vi "Supervisor Read Client.vi"() -> ()   [LabVIEW 2017]
uses:
  <vilib>/OPCUA/controls/NodeIds.ctl
  <vilib>/OPCUA/controls/NodeId.ctl
  <vilib>/OPCUA/NI OPC UA Client.lvlib
panel:
  in  "stop":bool
  out "error out":errorcluster
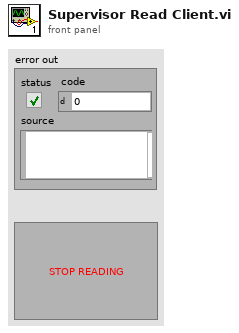
[diagram p1: front panel]
types:
  T1 = cluster{"message mode":enum16{"None", "Sign", "Sign and Encrypt"}, "security":enum16{"Basic256", "Basic128Rsa15"}}
  T2 = typedef "NodeIds.ctl" = T3[]
  T3 = typedef "NodeId.ctl" = string
  T4 = typedef "OPC UA Client Refnum.ctl" = refnum<k21>
  T5 = typedef "Subscription ID.ctl" = u32
  T6 = typedef "Subscription Data Change.ctl" = cluster{"node ID":T3, " value":variant, "timestamp":timestamp, "data type":T7, "status code":T8}
  T7 = typedef "Data Type.ctl" = u16
  T8 = typedef "OPC UA StatusCode.ctl" = u32
  T9 = cluster{"[0]":sgl, "[1]":sgl, "[2]":sgl, "[3]":sgl, "[4]":sgl, "[5]":sgl, "[6]":sgl, "[7]":sgl, "[8]":sgl, "[9]":sgl, "[10]":sgl, "[11]":sgl, "[12]":sgl, "[13]":sgl, "[14]":sgl, "[15]":sgl, "[16]":sgl, "[17]":sgl, "[18]":sgl, "[19]":sgl, "[20]":sgl, "[21]":sgl, "[22]":sgl, "[23]":sgl, "[24]":sgl, "[25]":sgl, "[26]":sgl, "[27]":sgl, "[28]":sgl, "[29]":sgl, "[30]":sgl, "[31]":sgl, "[32]":sgl, "[33]":sgl, "[34]":sgl, "[35]":sgl, "[36]":sgl, "[37]":sgl, "[38]":sgl, "[39]":sgl, "[40]":sgl, "[41]":sgl, "[42]":sgl, "[43]":sgl, "[44]":sgl, "[45]":sgl, "[46]":sgl, "[47]":sgl, "[48]":sgl, "[49]":sgl, "[50]":sgl, "[51]":sgl, "[52]":sgl, "[53]":sgl, "[54]":sgl, "[55]":sgl, "[56]":sgl, "[57]":sgl, "[58]":sgl, "[59]":sgl, "[60]":sgl, "[61]":sgl, "[62]":sgl}
  T10 = cluster{"[0]":sgl, "[1]":sgl, "[2]":sgl, "[3]":sgl, "[4]":sgl, "[5]":sgl, "[6]":sgl, "[7]":sgl, "[8]":sgl, "[9]":sgl}
  T11 = cluster{"[0]":bool, "[1]":bool, "[2]":bool, "[3]":bool, "[4]":bool, "[5]":bool, "[6]":bool, "[7]":bool, "[8]":bool, "[9]":bool, "[10]":bool, "[11]":bool, "[12]":bool, "[13]":bool, "[14]":bool, "[15]":bool, "[16]":bool, "[17]":bool, "[18]":bool, "[19]":bool, "[20]":bool, "[21]":bool, "[22]":bool, "[23]":bool, "[24]":bool, "[25]":bool, "[26]":bool, "[27]":bool, "[28]":bool, "[29]":bool, "[30]":bool, "[31]":bool, "[32]":bool, "[33]":bool, "[34]":bool, "[35]":bool, "[36]":bool, "[37]":bool, "[38]":bool, "[39]":bool, "[40]":bool, "[41]":bool, "[42]":bool, "[43]":bool, "[44]":bool, "[45]":bool, "[46]":bool, "[47]":bool, "[48]":bool, "[49]":bool, "[50]":bool, "[51]":bool, "[52]":bool, "[53]":bool, "[54]":bool, "[55]":bool, "[56]":bool, "[57]":bool, "[58]":bool, "[59]":bool, "[60]":bool, "[61]":bool, "[62]":bool}
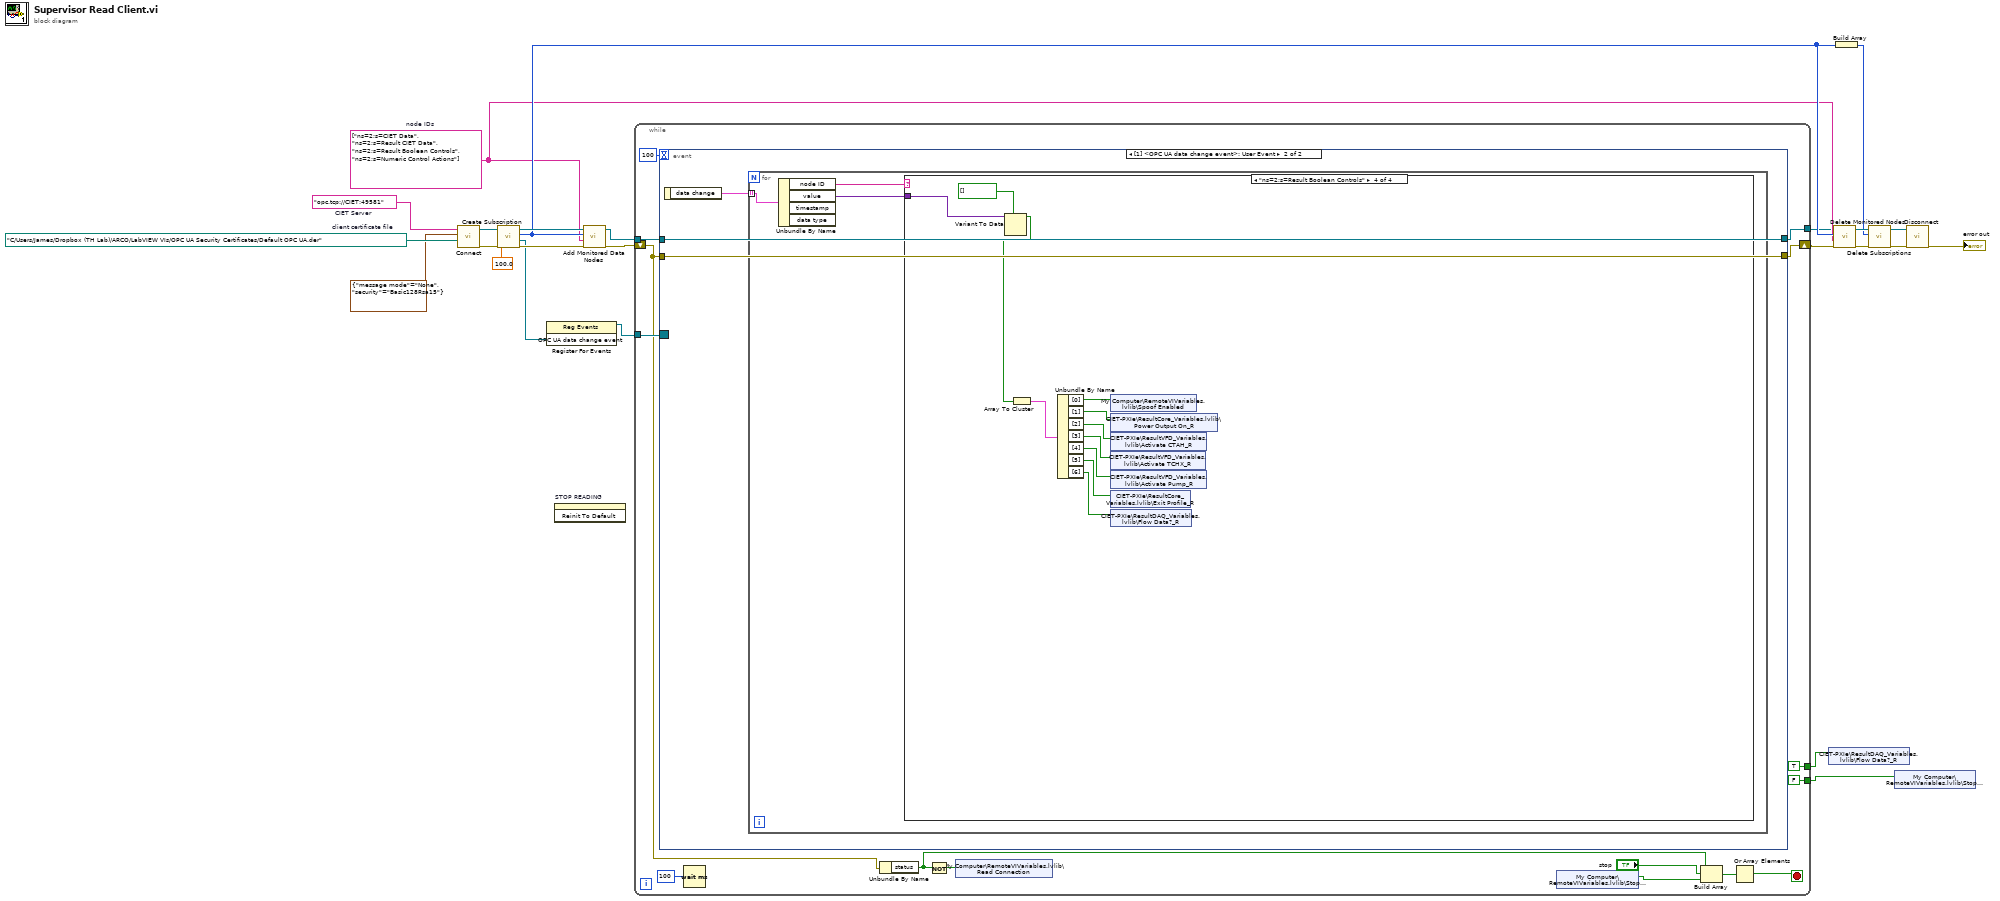
[diagram p0: block diagram]
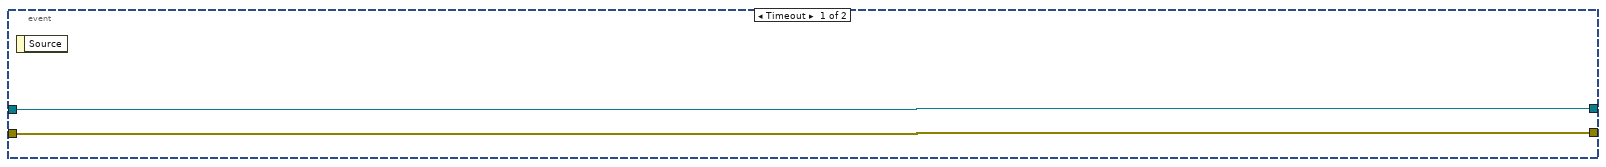
[diagram p2: hidden frame]
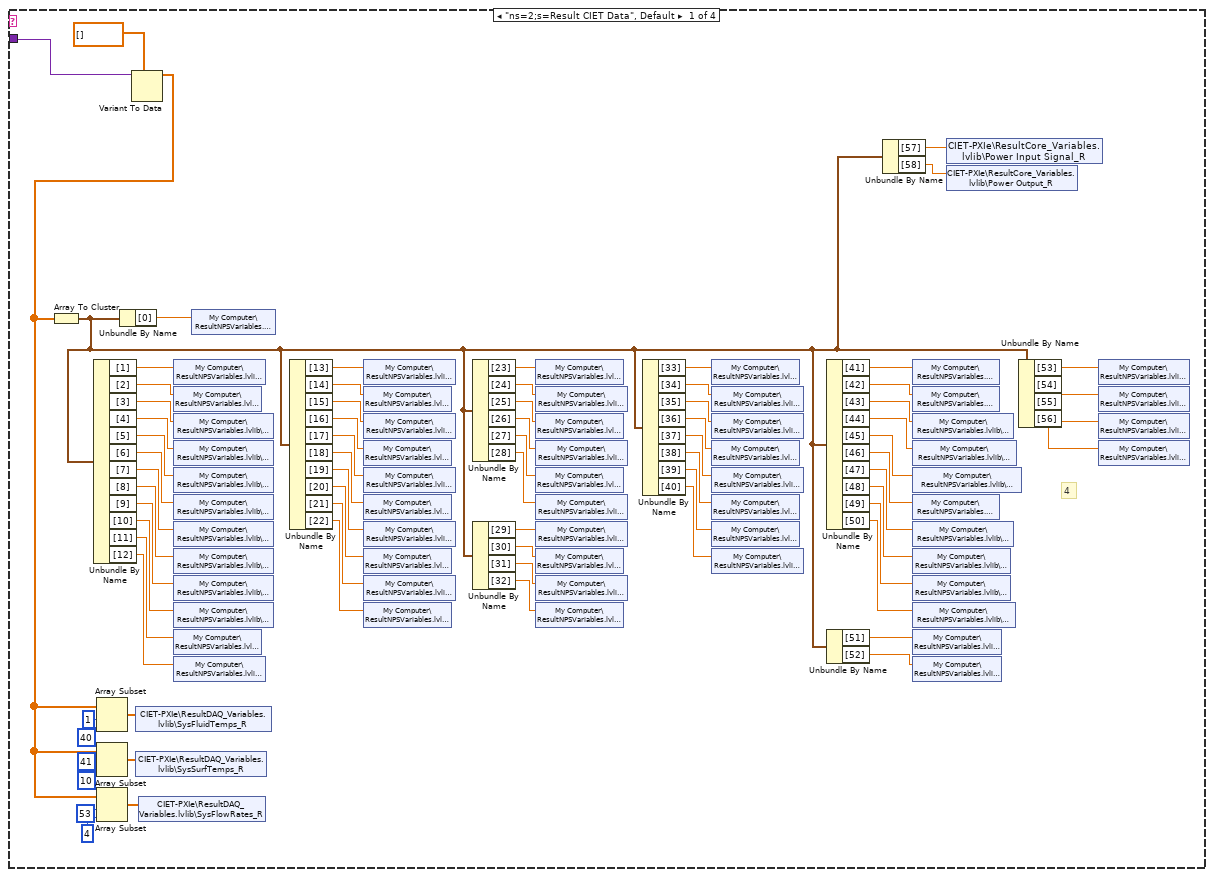
[diagram p3: hidden frame]
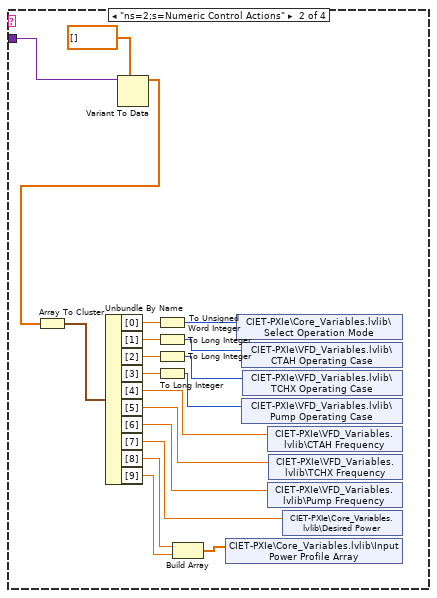
[diagram p4: hidden frame]
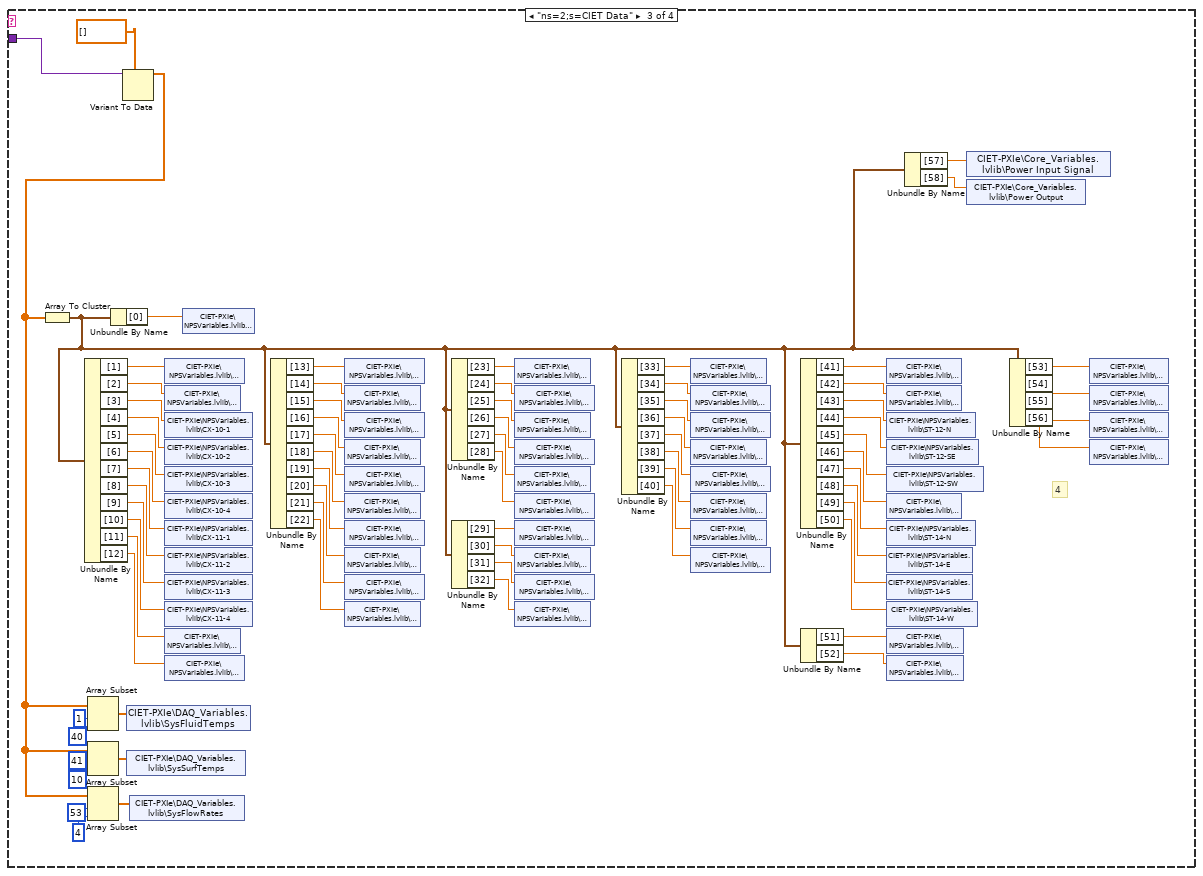
[diagram p5: hidden frame]
diagram:
  w7 = T2 ["ns=2;s=CIET Data", "ns=2;s=Result CIET Data", "ns=2;s=Result Boolean Controls", "ns=2;s=Numeric Control Actions"]  # node IDs
  w22 = path "C:/Users/James/Dropbox (TH Lab)/ARCO/LabVIEW VIs/OPC UA Security Certificates/Default OPC UA.der"  # client certificate file
  w23 = "opc.tcp://CIET:49581"  # CIET Server
  n1 = call <vilib>:"Connect.vi"("client certificate file"=w22, "security policy"=T1 {"message mode"=enum."None", "security"=enum."Basic128Rsa15"}, "server endpoint URL"=w23) -> ("error out"=w3:errorcluster, "OPC UA client refnum out"=w20:T4)  [unwired: 6 in, 1 out]
  n2 = call <vilib>:"Create Subscription.vi"("error in (no error)"=w3, "publishing interval (1000 ms)"=100.0, "OPC UA client refnum in"=w20) -> ("error out"=w18:errorcluster, "OPC UA data change event"=w17:refnum<user-event>, "subscription ID out"=w12:T5, "OPC UA client refnum out"=w19:T4)  [unwired: 4 in, 1 out]
  n3 = register-events(w17) -> (reference out=w10:refnum<event-registration>)  [unwired: 2 in, 1 out]
  n4 = invoke on="STOP READING" class="Bool" method="Reinit To Default"() -> ()  [unwired: 3 in, 3 out]
  n5 = call <vilib>:"Add Monitored Data Nodes.vi"("error in (no error)"=w18, "node IDs"=w7, "subscription ID in"=w12, "OPC UA client refnum in"=w19) -> ("error out"=w8:errorcluster, "OPC UA client refnum out"=w9:T4)  [unwired: 4 in, 2 out]
  n6 = while {
    tunnel: w10 -> [w39]
    tunnel: w9 -> [w38]
    tunnel: [w37] -> w6
    tunnel: [FALSE] -> w4
    shift-right: [w33] -> w2
    shift-left: w8 -> [w32]
    tunnel: [TRUE ("Flow Data?_R")] -> w1
    stop <- w31 stop-if-true
    n7 = event shown="[1] <OPC UA data change event>: User Event" {
      selector: w39 -> [_ _]
      dyn-events: _ -> [_ _]
      timeout: 100 -> [_ _]
      tunnel: w38 -> [w41 w44]
      tunnel: [w41 w44] -> w37
      tunnel: w32 -> [w40 w43]
      tunnel: [w40 w43] -> w33
      event Timeout {
        n8 = event-data() -> ()  [unwired: 1 in, 1 out]
      }
      event User Event {
        n9 = event-data() -> ("data change"=w42:T6[])  [unwired: 1 in]
        n10 = for {
          tunnel: w42 -> [w47] mode=indexing
          n11 = Unbundle By Name(w47) -> ("node ID"=w46:T3, "value"=w45:variant)  [unwired: 2 out]
          n12 = case shown="\"ns=2;s=Result Boolean Controls\"" w46 {
            tunnel: w45 -> [w53 w136 w151 w221]
            frame "ns=2;s=Result CIET Data", Default {
              # "4"
              n13 = Variant To Data(type=sgl[] [], Variant=w53) -> (data=w52:sgl[])  [unwired: 1 in, 1 out]
              n14 = Array To Cluster(array=w52) -> (cluster=w50:T9)
              n15 = Unbundle By Name(w50) -> ("[1]"=w60:sgl, "[2]"=w62:sgl, "[3]"=w63:sgl, "[4]"=w64:sgl, "[5]"=w65:sgl, "[6]"=w66:sgl, "[7]"=w67:sgl, "[8]"=w68:sgl, "[9]"=w69:sgl, "[10]"=w70:sgl, "[11]"=w71:sgl, "[12]"=w72:sgl)
              n16 = Array Subset(array=w52, index=1, length=40) -> (w117:sgl[])
              n17 = Array Subset(array=w52, index=41, length=10) -> (w118:sgl[])
              n18 = Array Subset(array=w52, index=53, length=4) -> (w119:sgl[])
              n19 = Unbundle By Name(w50) -> ("[0]"=w61:sgl)
              n20 = shared-variable "CIET-PXIe\\ResultDAQ_Variables.lvlib\\SysFluidTemps_R"(w117) -> ()  [unwired: 1 in, 1 out]
              n21 = shared-variable "CIET-PXIe\\ResultDAQ_Variables.lvlib\\SysSurfTemps_R"(w118) -> ()  [unwired: 1 in, 1 out]
              n22 = shared-variable "CIET-PXIe\\ResultDAQ_Variables.lvlib\\SysFlowRates_R"(w119) -> ()  [unwired: 1 in, 1 out]
              n23 = shared-variable "My Computer\\ResultNPSVariables.lvlib\\WT-10_R"(w60) -> ()  [unwired: 1 in, 1 out]
              n24 = shared-variable "My Computer\\ResultNPSVariables.lvlib\\BT-11_R"(w62) -> ()  [unwired: 1 in, 1 out]
              n25 = shared-variable "My Computer\\ResultNPSVariables.lvlib\\CX-10-1_R"(w63) -> ()  [unwired: 1 in, 1 out]
              n26 = shared-variable "My Computer\\ResultNPSVariables.lvlib\\CX-10-2_R"(w64) -> ()  [unwired: 1 in, 1 out]
              n27 = shared-variable "My Computer\\ResultNPSVariables.lvlib\\CX-10-3_R"(w65) -> ()  [unwired: 1 in, 1 out]
              n28 = shared-variable "My Computer\\ResultNPSVariables.lvlib\\CX-10-4_R"(w66) -> ()  [unwired: 1 in, 1 out]
              n29 = shared-variable "My Computer\\ResultNPSVariables.lvlib\\CX-11-1_R"(w67) -> ()  [unwired: 1 in, 1 out]
              n30 = shared-variable "My Computer\\ResultNPSVariables.lvlib\\CX-11-2_R"(w68) -> ()  [unwired: 1 in, 1 out]
              n31 = shared-variable "My Computer\\ResultNPSVariables.lvlib\\CX-11-3_R"(w69) -> ()  [unwired: 1 in, 1 out]
              n32 = shared-variable "My Computer\\ResultNPSVariables.lvlib\\CX-11-4_R"(w70) -> ()  [unwired: 1 in, 1 out]
              n33 = shared-variable "My Computer\\ResultNPSVariables.lvlib\\BT-12_R"(w71) -> ()  [unwired: 1 in, 1 out]
              n34 = shared-variable "My Computer\\ResultNPSVariables.lvlib\\WT-13_R"(w72) -> ()  [unwired: 1 in, 1 out]
              n35 = shared-variable "My Computer\\ResultNPSVariables.lvlib\\Time_R"(w61) -> ()  [unwired: 1 in, 1 out]
              n36 = Unbundle By Name(w50) -> ("[13]"=w73:sgl, "[14]"=w74:sgl, "[15]"=w75:sgl, "[16]"=w76:sgl, "[17]"=w77:sgl, "[18]"=w78:sgl, "[19]"=w79:sgl, "[20]"=w80:sgl, "[21]"=w81:sgl, "[22]"=w82:sgl)
              n37 = shared-variable "My Computer\\ResultNPSVariables.lvlib\\WT-20_R"(w73) -> ()  [unwired: 1 in, 1 out]
              n38 = shared-variable "My Computer\\ResultNPSVariables.lvlib\\BT-21_R"(w74) -> ()  [unwired: 1 in, 1 out]
              n39 = shared-variable "My Computer\\ResultNPSVariables.lvlib\\WT-22_R"(w75) -> ()  [unwired: 1 in, 1 out]
              n40 = shared-variable "My Computer\\ResultNPSVariables.lvlib\\BT-23_R"(w76) -> ()  [unwired: 1 in, 1 out]
              n41 = shared-variable "My Computer\\ResultNPSVariables.lvlib\\WT-24_R"(w77) -> ()  [unwired: 1 in, 1 out]
              n42 = shared-variable "My Computer\\ResultNPSVariables.lvlib\\BT-25_R"(w78) -> ()  [unwired: 1 in, 1 out]
              n43 = shared-variable "My Computer\\ResultNPSVariables.lvlib\\WT-26_R"(w79) -> ()  [unwired: 1 in, 1 out]
              n44 = shared-variable "My Computer\\ResultNPSVariables.lvlib\\BT-27_R"(w80) -> ()  [unwired: 1 in, 1 out]
              n45 = shared-variable "My Computer\\ResultNPSVariables.lvlib\\WT-28_R"(w81) -> ()  [unwired: 1 in, 1 out]
              n46 = shared-variable "My Computer\\ResultNPSVariables.lvlib\\BT-29_R"(w82) -> ()  [unwired: 1 in, 1 out]
              n47 = Unbundle By Name(w50) -> ("[23]"=w83:sgl, "[24]"=w84:sgl, "[25]"=w85:sgl, "[26]"=w86:sgl, "[27]"=w87:sgl, "[28]"=w88:sgl)
              n48 = Unbundle By Name(w50) -> ("[29]"=w89:sgl, "[30]"=w90:sgl, "[31]"=w91:sgl, "[32]"=w92:sgl)
              n49 = shared-variable "My Computer\\ResultNPSVariables.lvlib\\BT-30_R"(w83) -> ()  [unwired: 1 in, 1 out]
              n50 = shared-variable "My Computer\\ResultNPSVariables.lvlib\\WT-31_R"(w84) -> ()  [unwired: 1 in, 1 out]
              n51 = shared-variable "My Computer\\ResultNPSVariables.lvlib\\BT-32_R"(w85) -> ()  [unwired: 1 in, 1 out]
              n52 = shared-variable "My Computer\\ResultNPSVariables.lvlib\\WT-33_R"(w86) -> ()  [unwired: 1 in, 1 out]
              n53 = shared-variable "My Computer\\ResultNPSVariables.lvlib\\BT-34_R"(w87) -> ()  [unwired: 1 in, 1 out]
              n54 = shared-variable "My Computer\\ResultNPSVariables.lvlib\\WT-35_R"(w88) -> ()  [unwired: 1 in, 1 out]
              n55 = shared-variable "My Computer\\ResultNPSVariables.lvlib\\WT-40_R"(w89) -> ()  [unwired: 1 in, 1 out]
              n56 = shared-variable "My Computer\\ResultNPSVariables.lvlib\\BT-41_R"(w90) -> ()  [unwired: 1 in, 1 out]
              n57 = shared-variable "My Computer\\ResultNPSVariables.lvlib\\WT-42_R"(w91) -> ()  [unwired: 1 in, 1 out]
              n58 = shared-variable "My Computer\\ResultNPSVariables.lvlib\\BT-43_R"(w92) -> ()  [unwired: 1 in, 1 out]
              n59 = Unbundle By Name(w50) -> ("[33]"=w93:sgl, "[34]"=w94:sgl, "[35]"=w95:sgl, "[36]"=w96:sgl, "[37]"=w97:sgl, "[38]"=w98:sgl, "[39]"=w99:sgl, "[40]"=w100:sgl)
              n60 = shared-variable "My Computer\\ResultNPSVariables.lvlib\\BT-60_R"(w93) -> ()  [unwired: 1 in, 1 out]
              n61 = shared-variable "My Computer\\ResultNPSVariables.lvlib\\WT-61_R"(w94) -> ()  [unwired: 1 in, 1 out]
              n62 = shared-variable "My Computer\\ResultNPSVariables.lvlib\\WT-62_R"(w95) -> ()  [unwired: 1 in, 1 out]
              n63 = shared-variable "My Computer\\ResultNPSVariables.lvlib\\BT-63_R"(w96) -> ()  [unwired: 1 in, 1 out]
              n64 = shared-variable "My Computer\\ResultNPSVariables.lvlib\\WT-64_R"(w97) -> ()  [unwired: 1 in, 1 out]
              n65 = shared-variable "My Computer\\ResultNPSVariables.lvlib\\BT-65_R"(w98) -> ()  [unwired: 1 in, 1 out]
              n66 = shared-variable "My Computer\\ResultNPSVariables.lvlib\\BT-66_R"(w99) -> ()  [unwired: 1 in, 1 out]
              n67 = shared-variable "My Computer\\ResultNPSVariables.lvlib\\WT-67_R"(w100) -> ()  [unwired: 1 in, 1 out]
              n68 = Unbundle By Name(w50) -> ("[41]"=w101:sgl, "[42]"=w102:sgl, "[43]"=w103:sgl, "[44]"=w104:sgl, "[45]"=w105:sgl, "[46]"=w106:sgl, "[47]"=w107:sgl, "[48]"=w108:sgl, "[49]"=w109:sgl, "[50]"=w110:sgl)
              n69 = Unbundle By Name(w50) -> ("[51]"=w111:sgl, "[52]"=w112:sgl)
              n70 = Unbundle By Name(w50) -> ("[57]"=w49:sgl, "[58]"=w48:sgl)
              n71 = shared-variable "My Computer\\ResultNPSVariables.lvlib\\ST-10_R"(w101) -> ()  [unwired: 1 in, 1 out]
              n72 = shared-variable "My Computer\\ResultNPSVariables.lvlib\\ST-11_R"(w102) -> ()  [unwired: 1 in, 1 out]
              n73 = shared-variable "My Computer\\ResultNPSVariables.lvlib\\ST-12-N_R"(w103) -> ()  [unwired: 1 in, 1 out]
              n74 = shared-variable "My Computer\\ResultNPSVariables.lvlib\\ST-12-SE_R"(w104) -> ()  [unwired: 1 in, 1 out]
              n75 = shared-variable "My Computer\\ResultNPSVariables.lvlib\\ST-12-SW_R"(w105) -> ()  [unwired: 1 in, 1 out]
              n76 = shared-variable "My Computer\\ResultNPSVariables.lvlib\\ST-13_R"(w106) -> ()  [unwired: 1 in, 1 out]
              n77 = shared-variable "My Computer\\ResultNPSVariables.lvlib\\ST-14-N_R"(w107) -> ()  [unwired: 1 in, 1 out]
              n78 = shared-variable "My Computer\\ResultNPSVariables.lvlib\\ST-14-E_R"(w108) -> ()  [unwired: 1 in, 1 out]
              n79 = shared-variable "My Computer\\ResultNPSVariables.lvlib\\ST-14-S_R"(w109) -> ()  [unwired: 1 in, 1 out]
              n80 = shared-variable "My Computer\\ResultNPSVariables.lvlib\\ST-14-W_R"(w110) -> ()  [unwired: 1 in, 1 out]
              n81 = shared-variable "My Computer\\ResultNPSVariables.lvlib\\AT-01_R"(w111) -> ()  [unwired: 1 in, 1 out]
              n82 = shared-variable "My Computer\\ResultNPSVariables.lvlib\\AT-02_R"(w112) -> ()  [unwired: 1 in, 1 out]
              n83 = shared-variable "CIET-PXIe\\ResultCore_Variables.lvlib\\Power Input Signal_R"(w49) -> ()  [unwired: 1 in, 1 out]
              n84 = shared-variable "CIET-PXIe\\ResultCore_Variables.lvlib\\Power Output_R"(w48) -> ()  [unwired: 1 in, 1 out]
              n85 = Unbundle By Name(w50) -> ("[53]"=w113:sgl, "[54]"=w114:sgl, "[55]"=w115:sgl, "[56]"=w116:sgl)
              n86 = shared-variable "My Computer\\ResultNPSVariables.lvlib\\FM-20_R"(w113) -> ()  [unwired: 1 in, 1 out]
              n87 = shared-variable "My Computer\\ResultNPSVariables.lvlib\\FM-30_R"(w114) -> ()  [unwired: 1 in, 1 out]
              n88 = shared-variable "My Computer\\ResultNPSVariables.lvlib\\FM-40_R"(w115) -> ()  [unwired: 1 in, 1 out]
              n89 = shared-variable "My Computer\\ResultNPSVariables.lvlib\\FM-60_R"(w116) -> ()  [unwired: 1 in, 1 out]
            }
            frame "ns=2;s=Numeric Control Actions" {
              n90 = Variant To Data(type=sgl[] [], Variant=w136) -> (data=w138:sgl[])  [unwired: 1 in, 1 out]
              n91 = Array To Cluster(array=w138) -> (cluster=w137:T10)
              n92 = Unbundle By Name(w137) -> ("[0]"=w134:sgl, "[1]"=w133:sgl, "[2]"=w132:sgl, "[3]"=w131:sgl, "[4]"=w126:sgl, "[5]"=w125:sgl, "[6]"=w124:sgl, "[7]"=w123:sgl, "[8]"=w121:sgl, "[9]"=w120:sgl)
              n93 = To Unsigned Word Integer(number=w134) -> (unsigned 16bit integer=w130:u16)
              n94 = To Long Integer(number=w133) -> (32bit integer=w129:i32)
              n95 = To Long Integer(number=w132) -> (32bit integer=w128:i32)
              n96 = To Long Integer(number=w131) -> (32bit integer=w127:i32)
              n97 = Build Array(w121, w120) -> (w122:sgl[])
              n98 = shared-variable "CIET-PXIe\\Core_Variables.lvlib\\Input Power Profile Array"(w122) -> ()  [unwired: 1 in, 1 out]
              n99 = shared-variable "CIET-PXIe\\Core_Variables.lvlib\\Select Operation Mode"(w130) -> ()  [unwired: 1 in, 1 out]
              n100 = shared-variable "CIET-PXIe\\VFD_Variables.lvlib\\CTAH Operating Case"(w129) -> ()  [unwired: 1 in, 1 out]
              n101 = shared-variable "CIET-PXIe\\VFD_Variables.lvlib\\Pump Operating Case"(w127) -> ()  [unwired: 1 in, 1 out]
              n102 = shared-variable "CIET-PXIe\\VFD_Variables.lvlib\\TCHX Operating Case"(w128) -> ()  [unwired: 1 in, 1 out]
              n103 = shared-variable "CIET-PXIe\\VFD_Variables.lvlib\\CTAH Frequency"(w126) -> ()  [unwired: 1 in, 1 out]
              n104 = shared-variable "CIET-PXIe\\VFD_Variables.lvlib\\Pump Frequency"(w124) -> ()  [unwired: 1 in, 1 out]
              n105 = shared-variable "CIET-PXIe\\VFD_Variables.lvlib\\TCHX Frequency"(w125) -> ()  [unwired: 1 in, 1 out]
              n106 = shared-variable "CIET-PXIe\\Core_Variables.lvlib\\Desired Power"(w123) -> ()  [unwired: 1 in, 1 out]
            }
            frame "ns=2;s=CIET Data" {
              # "4"
              n107 = Variant To Data(type=sgl[] [], Variant=w151) -> (data=w148:sgl[])  [unwired: 1 in, 1 out]
              n108 = Array To Cluster(array=w148) -> (cluster=w141:T9)
              n109 = Unbundle By Name(w141) -> ("[1]"=w150:sgl, "[2]"=w153:sgl, "[3]"=w154:sgl, "[4]"=w155:sgl, "[5]"=w156:sgl, "[6]"=w157:sgl, "[7]"=w158:sgl, "[8]"=w159:sgl, "[9]"=w160:sgl, "[10]"=w161:sgl, "[11]"=w162:sgl, "[12]"=w163:sgl)
              n110 = Array Subset(array=w148, index=1, length=40) -> (w208:sgl[])
              n111 = Array Subset(array=w148, index=41, length=10) -> (w209:sgl[])
              n112 = Array Subset(array=w148, index=53, length=4) -> (w210:sgl[])
              n113 = Unbundle By Name(w141) -> ("[0]"=w152:sgl)
              n114 = shared-variable "CIET-PXIe\\DAQ_Variables.lvlib\\SysFluidTemps"(w208) -> ()  [unwired: 1 in, 1 out]
              n115 = shared-variable "CIET-PXIe\\DAQ_Variables.lvlib\\SysSurfTemps"(w209) -> ()  [unwired: 1 in, 1 out]
              n116 = shared-variable "CIET-PXIe\\DAQ_Variables.lvlib\\SysFlowRates"(w210) -> ()  [unwired: 1 in, 1 out]
              n117 = shared-variable "CIET-PXIe\\NPSVariables.lvlib\\WT-10"(w150) -> ()  [unwired: 1 in, 1 out]
              n118 = shared-variable "CIET-PXIe\\NPSVariables.lvlib\\BT-11"(w153) -> ()  [unwired: 1 in, 1 out]
              n119 = shared-variable "CIET-PXIe\\NPSVariables.lvlib\\CX-10-1"(w154) -> ()  [unwired: 1 in, 1 out]
              n120 = shared-variable "CIET-PXIe\\NPSVariables.lvlib\\CX-10-2"(w155) -> ()  [unwired: 1 in, 1 out]
              n121 = shared-variable "CIET-PXIe\\NPSVariables.lvlib\\CX-10-3"(w156) -> ()  [unwired: 1 in, 1 out]
              n122 = shared-variable "CIET-PXIe\\NPSVariables.lvlib\\CX-10-4"(w157) -> ()  [unwired: 1 in, 1 out]
              n123 = shared-variable "CIET-PXIe\\NPSVariables.lvlib\\CX-11-1"(w158) -> ()  [unwired: 1 in, 1 out]
              n124 = shared-variable "CIET-PXIe\\NPSVariables.lvlib\\CX-11-2"(w159) -> ()  [unwired: 1 in, 1 out]
              n125 = shared-variable "CIET-PXIe\\NPSVariables.lvlib\\CX-11-3"(w160) -> ()  [unwired: 1 in, 1 out]
              n126 = shared-variable "CIET-PXIe\\NPSVariables.lvlib\\CX-11-4"(w161) -> ()  [unwired: 1 in, 1 out]
              n127 = shared-variable "CIET-PXIe\\NPSVariables.lvlib\\BT-12"(w162) -> ()  [unwired: 1 in, 1 out]
              n128 = shared-variable "CIET-PXIe\\NPSVariables.lvlib\\WT-13"(w163) -> ()  [unwired: 1 in, 1 out]
              n129 = shared-variable "CIET-PXIe\\NPSVariables.lvlib\\Time"(w152) -> ()  [unwired: 1 in, 1 out]
              n130 = Unbundle By Name(w141) -> ("[13]"=w164:sgl, "[14]"=w165:sgl, "[15]"=w166:sgl, "[16]"=w167:sgl, "[17]"=w168:sgl, "[18]"=w169:sgl, "[19]"=w170:sgl, "[20]"=w171:sgl, "[21]"=w172:sgl, "[22]"=w173:sgl)
              n131 = shared-variable "CIET-PXIe\\NPSVariables.lvlib\\WT-20"(w164) -> ()  [unwired: 1 in, 1 out]
              n132 = shared-variable "CIET-PXIe\\NPSVariables.lvlib\\BT-21"(w165) -> ()  [unwired: 1 in, 1 out]
              n133 = shared-variable "CIET-PXIe\\NPSVariables.lvlib\\WT-22"(w166) -> ()  [unwired: 1 in, 1 out]
              n134 = shared-variable "CIET-PXIe\\NPSVariables.lvlib\\BT-23"(w167) -> ()  [unwired: 1 in, 1 out]
              n135 = shared-variable "CIET-PXIe\\NPSVariables.lvlib\\WT-24"(w168) -> ()  [unwired: 1 in, 1 out]
              n136 = shared-variable "CIET-PXIe\\NPSVariables.lvlib\\BT-25"(w169) -> ()  [unwired: 1 in, 1 out]
              n137 = shared-variable "CIET-PXIe\\NPSVariables.lvlib\\WT-26"(w170) -> ()  [unwired: 1 in, 1 out]
              n138 = shared-variable "CIET-PXIe\\NPSVariables.lvlib\\BT-27"(w171) -> ()  [unwired: 1 in, 1 out]
              n139 = shared-variable "CIET-PXIe\\NPSVariables.lvlib\\WT-28"(w172) -> ()  [unwired: 1 in, 1 out]
              n140 = shared-variable "CIET-PXIe\\NPSVariables.lvlib\\BT-29"(w173) -> ()  [unwired: 1 in, 1 out]
              n141 = Unbundle By Name(w141) -> ("[23]"=w174:sgl, "[24]"=w175:sgl, "[25]"=w176:sgl, "[26]"=w177:sgl, "[27]"=w178:sgl, "[28]"=w179:sgl)
              n142 = Unbundle By Name(w141) -> ("[29]"=w180:sgl, "[30]"=w181:sgl, "[31]"=w182:sgl, "[32]"=w183:sgl)
              n143 = shared-variable "CIET-PXIe\\NPSVariables.lvlib\\BT-30"(w174) -> ()  [unwired: 1 in, 1 out]
              n144 = shared-variable "CIET-PXIe\\NPSVariables.lvlib\\WT-31"(w175) -> ()  [unwired: 1 in, 1 out]
              n145 = shared-variable "CIET-PXIe\\NPSVariables.lvlib\\BT-32"(w176) -> ()  [unwired: 1 in, 1 out]
              n146 = shared-variable "CIET-PXIe\\NPSVariables.lvlib\\WT-33"(w177) -> ()  [unwired: 1 in, 1 out]
              n147 = shared-variable "CIET-PXIe\\NPSVariables.lvlib\\BT-34"(w178) -> ()  [unwired: 1 in, 1 out]
              n148 = shared-variable "CIET-PXIe\\NPSVariables.lvlib\\WT-35"(w179) -> ()  [unwired: 1 in, 1 out]
              n149 = shared-variable "CIET-PXIe\\NPSVariables.lvlib\\WT-40"(w180) -> ()  [unwired: 1 in, 1 out]
              n150 = shared-variable "CIET-PXIe\\NPSVariables.lvlib\\BT-41"(w181) -> ()  [unwired: 1 in, 1 out]
              n151 = shared-variable "CIET-PXIe\\NPSVariables.lvlib\\WT-42"(w182) -> ()  [unwired: 1 in, 1 out]
              n152 = shared-variable "CIET-PXIe\\NPSVariables.lvlib\\BT-43"(w183) -> ()  [unwired: 1 in, 1 out]
              n153 = Unbundle By Name(w141) -> ("[33]"=w184:sgl, "[34]"=w185:sgl, "[35]"=w186:sgl, "[36]"=w187:sgl, "[37]"=w188:sgl, "[38]"=w189:sgl, "[39]"=w190:sgl, "[40]"=w191:sgl)
              n154 = shared-variable "CIET-PXIe\\NPSVariables.lvlib\\BT-60"(w184) -> ()  [unwired: 1 in, 1 out]
              n155 = shared-variable "CIET-PXIe\\NPSVariables.lvlib\\WT-61"(w185) -> ()  [unwired: 1 in, 1 out]
              n156 = shared-variable "CIET-PXIe\\NPSVariables.lvlib\\WT-62"(w186) -> ()  [unwired: 1 in, 1 out]
              n157 = shared-variable "CIET-PXIe\\NPSVariables.lvlib\\BT-63"(w187) -> ()  [unwired: 1 in, 1 out]
              n158 = shared-variable "CIET-PXIe\\NPSVariables.lvlib\\WT-64"(w188) -> ()  [unwired: 1 in, 1 out]
              n159 = shared-variable "CIET-PXIe\\NPSVariables.lvlib\\BT-65"(w189) -> ()  [unwired: 1 in, 1 out]
              n160 = shared-variable "CIET-PXIe\\NPSVariables.lvlib\\BT-66"(w190) -> ()  [unwired: 1 in, 1 out]
              n161 = shared-variable "CIET-PXIe\\NPSVariables.lvlib\\WT-67"(w191) -> ()  [unwired: 1 in, 1 out]
              n162 = Unbundle By Name(w141) -> ("[41]"=w192:sgl, "[42]"=w193:sgl, "[43]"=w194:sgl, "[44]"=w195:sgl, "[45]"=w196:sgl, "[46]"=w197:sgl, "[47]"=w198:sgl, "[48]"=w199:sgl, "[49]"=w200:sgl, "[50]"=w201:sgl)
              n163 = Unbundle By Name(w141) -> ("[51]"=w202:sgl, "[52]"=w203:sgl)
              n164 = shared-variable "CIET-PXIe\\NPSVariables.lvlib\\ST-10"(w192) -> ()  [unwired: 1 in, 1 out]
              n165 = shared-variable "CIET-PXIe\\NPSVariables.lvlib\\ST-11"(w193) -> ()  [unwired: 1 in, 1 out]
              n166 = shared-variable "CIET-PXIe\\NPSVariables.lvlib\\ST-12-N"(w194) -> ()  [unwired: 1 in, 1 out]
              n167 = shared-variable "CIET-PXIe\\NPSVariables.lvlib\\ST-12-SE"(w195) -> ()  [unwired: 1 in, 1 out]
              n168 = shared-variable "CIET-PXIe\\NPSVariables.lvlib\\ST-12-SW"(w196) -> ()  [unwired: 1 in, 1 out]
              n169 = shared-variable "CIET-PXIe\\NPSVariables.lvlib\\ST-13"(w197) -> ()  [unwired: 1 in, 1 out]
              n170 = shared-variable "CIET-PXIe\\NPSVariables.lvlib\\ST-14-N"(w198) -> ()  [unwired: 1 in, 1 out]
              n171 = shared-variable "CIET-PXIe\\NPSVariables.lvlib\\ST-14-E"(w199) -> ()  [unwired: 1 in, 1 out]
              n172 = shared-variable "CIET-PXIe\\NPSVariables.lvlib\\ST-14-S"(w200) -> ()  [unwired: 1 in, 1 out]
              n173 = shared-variable "CIET-PXIe\\NPSVariables.lvlib\\ST-14-W"(w201) -> ()  [unwired: 1 in, 1 out]
              n174 = shared-variable "CIET-PXIe\\NPSVariables.lvlib\\AT-01"(w202) -> ()  [unwired: 1 in, 1 out]
              n175 = shared-variable "CIET-PXIe\\NPSVariables.lvlib\\AT-02"(w203) -> ()  [unwired: 1 in, 1 out]
              n176 = Unbundle By Name(w141) -> ("[57]"=w140:sgl, "[58]"=w139:sgl)
              n177 = shared-variable "CIET-PXIe\\Core_Variables.lvlib\\Power Input Signal"(w140) -> ()  [unwired: 1 in, 1 out]
              n178 = shared-variable "CIET-PXIe\\Core_Variables.lvlib\\Power Output"(w139) -> ()  [unwired: 1 in, 1 out]
              n179 = Unbundle By Name(w141) -> ("[53]"=w204:sgl, "[54]"=w205:sgl, "[55]"=w206:sgl, "[56]"=w207:sgl)
              n180 = shared-variable "CIET-PXIe\\NPSVariables.lvlib\\FM-20"(w204) -> ()  [unwired: 1 in, 1 out]
              n181 = shared-variable "CIET-PXIe\\NPSVariables.lvlib\\FM-30"(w205) -> ()  [unwired: 1 in, 1 out]
              n182 = shared-variable "CIET-PXIe\\NPSVariables.lvlib\\FM-40"(w206) -> ()  [unwired: 1 in, 1 out]
              n183 = shared-variable "CIET-PXIe\\NPSVariables.lvlib\\FM-60"(w207) -> ()  [unwired: 1 in, 1 out]
            }
            frame "ns=2;s=Result Boolean Controls" {
              n184 = Variant To Data(type=bool[] [], Variant=w221) -> (data=w219:bool[])  [unwired: 1 in, 1 out]
              n185 = Array To Cluster(array=w219) -> (cluster=w218:T11)
              n186 = Unbundle By Name(w218) -> ("[0]"=w217:bool, "[1]"=w216:bool, "[2]"=w215:bool, "[3]"=w214:bool, "[4]"=w213:bool, "[5]"=w212:bool, "[6]"=w211:bool)
              n187 = shared-variable "My Computer\\RemoteVIVariables.lvlib\\Spoof Enabled"(w217) -> ()  [unwired: 1 in, 1 out]
              n188 = shared-variable "CIET-PXIe\\ResultCore_Variables.lvlib\\Power Output On_R"(w216) -> ()  [unwired: 1 in, 1 out]
              n189 = shared-variable "CIET-PXIe\\ResultVFD_Variables.lvlib\\Activate CTAH_R"(w215) -> ()  [unwired: 1 in, 1 out]
              n190 = shared-variable "CIET-PXIe\\ResultVFD_Variables.lvlib\\Activate TCHX_R"(w214) -> ()  [unwired: 1 in, 1 out]
              n191 = shared-variable "CIET-PXIe\\ResultVFD_Variables.lvlib\\Activate Pump_R"(w213) -> ()  [unwired: 1 in, 1 out]
              n192 = shared-variable "CIET-PXIe\\ResultCore_Variables.lvlib\\Exit Profile_R"(w212) -> ()  [unwired: 1 in, 1 out]
              n193 = shared-variable "CIET-PXIe\\ResultDAQ_Variables.lvlib\\Flow Data?_R"(w211) -> ()  [unwired: 1 in, 1 out]
            }
          }
        }
      }
    }
    n194 = Wait (ms)(milliseconds to wait=u32 100 ("millisecond timer value")) -> ()  [unwired: 1 out]
    n195 = Unbundle By Name(w32) -> ("status"=w27:bool)
    n196 = Not(x=w27) -> (.not. x?=w34:bool)
    n197 = shared-variable "My Computer\\RemoteVIVariables.lvlib\\Read Connection"(w34) -> ()  [unwired: 1 in, 1 out]
    n198 = shared-variable "My Computer\\RemoteVIVariables.lvlib\\Stop Reading"() -> (w30:bool)  [unwired: 1 in, 1 out]
    n199 = Build Array(w27, "stop", w30) -> (w28:bool[])
    n200 = Or Array Elements(Boolean array=w28) -> (logical OR=w31:bool)
  }
  n201 = shared-variable "CIET-PXIe\\ResultDAQ_Variables.lvlib\\Flow Data?_R"(w1) -> ()  [unwired: 1 in, 1 out]
  n202 = call <vilib>:"Delete Monitored Nodes.vi"("error in (no error)"=w2, "node IDs"=w7, "subscription ID in"=w12, "OPC UA client refnum in"=w6) -> ("error out"=w13:errorcluster, "OPC UA client refnum out"=w14:T4)  [unwired: 3 in, 3 out]
  n203 = Build Array(w12) -> (w11:T5[])
  n204 = call <vilib>:"Delete Subscriptions.vi"("error in (no error)"=w13, "subscription IDs"=w11, "OPC UA client refnum in"=w14) -> ("error out"=w15:errorcluster, "OPC UA client refnum out"=w16:T4)  [unwired: 6 in, 1 out]
  n205 = shared-variable "My Computer\\RemoteVIVariables.lvlib\\Stop Reading"(w4) -> ()  [unwired: 1 in, 1 out]
  n206 = call <vilib>:"Disconnect.vi"("error in (no error)"=w15, "OPC UA client refnum in"=w16) -> ("error out"=→"error out":errorcluster)  [unwired: 9 in]
